vi "SubProcessEngine.GetNextState.vi"(8 "error in (no error)":errorcluster, 9 "State":T3, 10 "timeout in ms (5)":i32=5, 11 "Q":refnum<queue>) -> (0 "error out":errorcluster, 1 "State":T3, 2 "timed out?":bool, 3 "Data":T1={"Cmd"=enum."Publish", "Parameters"=variant})   [LabVIEW 2025, in "XNET Bus Monitor Client.lvlib"]
uses:
  XNET Bus Monitor Client.lvlib
  Types/SubProcessEngine.State.ctl
  Types/SubProcessEngine.CmdQueueData.ctl
  Types/SubProcessEngine.CmdQueueData.Cmd.ctl
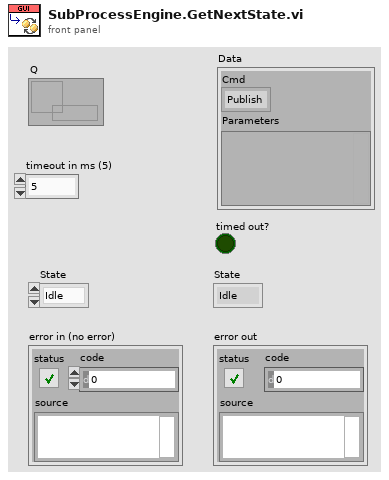
[diagram p1: front panel]
types:
  T1 = typedef "XNET Bus Monitor Client.lvlib/SubProcessEngine.CmdQueueData.ctl" = cluster{"Cmd":T2, "Parameters":variant}
  T2 = typedef "XNET Bus Monitor Client.lvlib/SubProcessEngine.CmdQueueData.Cmd.ctl" = enum16{"Arm", "Publish", "Stop", "Exit"}
  T3 = typedef "XNET Bus Monitor Client.lvlib/SubProcessEngine.State.ctl" = enum8{"Idle", "Arm", "Process", "Stop", "Exit"}
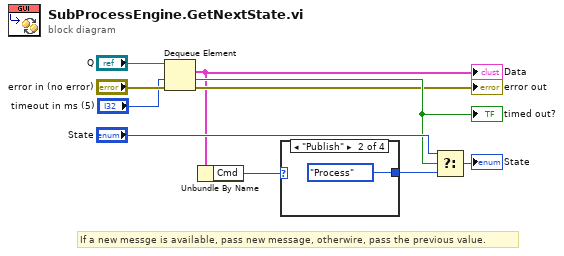
[diagram p0: block diagram]
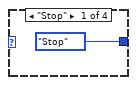
[diagram p2: hidden frame]
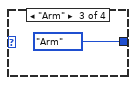
[diagram p3: hidden frame]
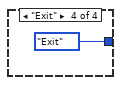
[diagram p4: hidden frame]
diagram:
  # "If a new messge is available, pass new message, otherwire, pass the previous value."
  n1 = Dequeue Element(queue="Q", timeout in ms (-1)="timeout in ms (5)", error in (no error)="error in (no error)") -> (element=w3:T1, timed out?=w7:bool, error out=→"error out":errorcluster)  [unwired: 1 out]
  "Data" <- w3
  "timed out?" <- w7
  n2 = Unbundle By Name(w3) -> ("Cmd"=w2:T2)
  n3 = case shown="\"Publish\"" w2 {
    tunnel: [SubProcessEngine.State."Stop" ("State") SubProcessEngine.State."Process" ("State") SubProcessEngine.State."Arm" ("State") SubProcessEngine.State."Exit" ("State")] -> w1
    frame "Stop" {
    }
    frame "Publish" {
    }
    frame "Arm" {
    }
    frame "Exit" {
    }
  }
  n4 = Select(t="State", s=w7, f=w1) -> (s? t:f=→"State":T3)
